vi "Keithley 27XX Math Measurement.vi"() -> ()   [LabVIEW 2020]
doc: "This VI shows how to use the Math Calculation feature with a single point measurement."
uses:
  <instrlib>/Keithley 27XX/Public/Data/Read Single Point.vi
  <instrlib>/Keithley 27XX/Keithley 27XX.lvlib
panel:
  in  "Serial Configuration":T1={"Baud Rate (9600)"=9600, "Flow Control (1: XON/XOFF)"=1, "Termination Char (0:CR)"=0} {"Termination Char (0:CR)" items=["CR", "LF"]; "Flow Control (1: XON/XOFF)" items=["None", "XON/XOFF", "RTS/CTS (2701 Only)", "XON/XOFF & RTS/CTS (2701 Only)"]; "Baud Rate (9600)" items=["300"=300, "600"=600, "1200"=1200, "2400"=2400, "4800"=4800, "9600"=9600, "19.2k"=19200, "38.4k (2701 Only)"=38400, "57.6k (2701 Only)"=57600, "115.2k (2701 Only)"=115200]}
  in  "Channel List (101)":string="101"
  in  "Offset (0)":dbl
  in  "Scalar (1)":dbl=1.0
  in  "VISA resource name":refnum<visa-resource-name>
  in  "Function (0: DC Voltage)":u16(ring) items=["DC Voltage", "AC Voltage", "DC Current", "AC Current", "Resistance", "Four-Wire Resistance", "Temperature (C)", "Frequency", "Period", "Continuity"]
  out "Measurement Data":dbl
  # "© 2005 National Instruments Corporation.  ALL RIGHTS RESERVED."
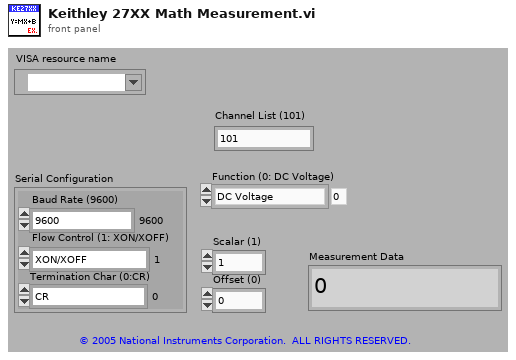
[diagram p1: front panel]
types:
  T1 = cluster{"Baud Rate (9600)":u32, "Flow Control (1: XON/XOFF)":u16, "Termination Char (0:CR)":u16}
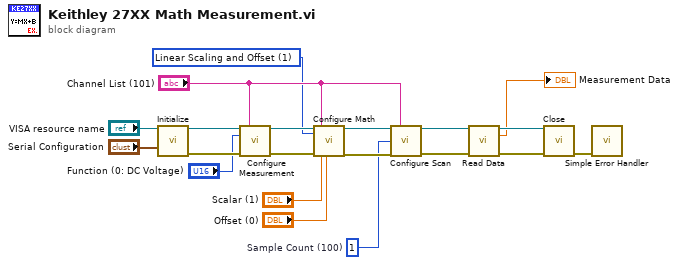
[diagram p0: block diagram]
diagram:
  w4 = 1  # Sample Count (100)
  w2 = u16 1 items=["None", "Linear Scaling and Offset", "Percent", "Reciprocal"] ("Math Format (2: Percent)")
  n1 = call <instrlib>:"Initialize.vi"("VISA resource name"="VISA resource name", "Serial Configuration"="Serial Configuration") -> ("VISA resource name out"=w20:refnum<visa-resource-name>, "error out"=w19:errorcluster)  [unwired: 12 in]
  n2 = call <instrlib>:"Configure Measurement.vi"("VISA resource name"=w20, "Scan List (Empty)"="Channel List (101)", "Function (0: DC Voltage)"="Function (0: DC Voltage)", "error in (no error)"=w19) -> ("VISA resource name out"=w13:refnum<visa-resource-name>, "error out"=w12:errorcluster)  [unwired: 10 in]
  n3 = call <instrlib>:"Configure Math.vi"("VISA resource name"=w13, "Math Format (2: Percent)"=w2, "error in (no error)"=w12, "Channel List (Empty)"="Channel List (101)", "Scalar (1)"="Scalar (1)", "Offset (0)"="Offset (0)") -> ("VISA resource name out"=w9:refnum<visa-resource-name>, "error out"=w6:errorcluster)  [unwired: 12 in]
  n4 = call <instrlib>:"Configure Scan.vi"("VISA resource name"=w9, "Channel List (101:110)"="Channel List (101)", "Sample Count (100)"=w4, "error in (no error)"=w6) -> ("VISA resource name out"=w8:refnum<visa-resource-name>, "error out"=w7:errorcluster)  [unwired: 10 in]
  n5 = call-poly <instrlib>:"Read Data.vi"("VISA resource name"=w8, "error in (no error)"=w7) -> ("VISA resource name out"=w16:refnum<visa-resource-name>, "Measurement Data"=→"Measurement Data":dbl, "error out"=w15:errorcluster)  [unwired: 11 in]
  n6 = call <instrlib>:"Close.vi"("VISA resource name"=w16, "error in (no error)"=w15) -> ("error out"=w14:errorcluster)  [unwired: 13 in]
  n7 = call <vilib>:"Simple Error Handler.vi"("error in (no error)"=w14) -> ()  [unwired: 4 in, 5 out]
